vi "Global 1.vi"() -> ()   [LabVIEW 2015]
panel:
  in  "error in (no error)":errorcluster
  in  "DAQmx Device Name":tag
  in  "Acq Time [ms]":dbl
  in  "Frequency [Hz]":dbl
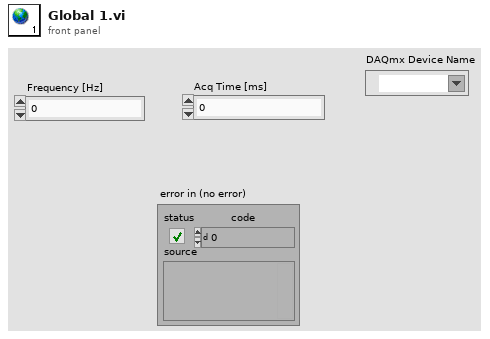
[diagram p1: front panel]
diagram:
